vi "DatabaseHand_Element_Get(string).vi"(7 "nd queue":bool, 8 "error in (no error)":errorcluster, 9 "default value":string, 10 "name":string, 11 "Database RefNum in":T1) -> (0 "error out":errorcluster, 1 "type":string, 2 "value":string, 3 "Database RefNum out":T1, 4 "permissions":string="RW", 5 "group":string, 6 "unit":string)   [LabVIEW 2016]
doc: "This VI finds the RefNum of an existing object with the input Name or creates a new object if the Name is not found or Name is unwired or an empty string.\nCopyright 2001 VI Engineering, Inc."
uses:
  DatabaseHand_RefNum.ctl
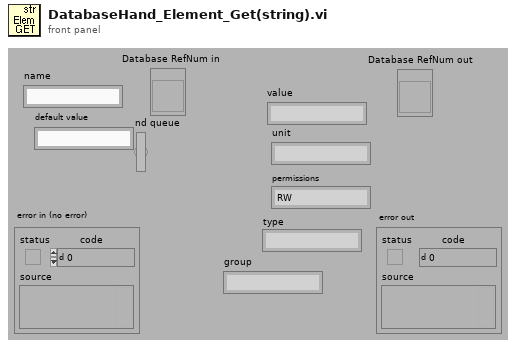
[diagram p1: front panel]
types:
  T1 = typedef "DatabaseHand_RefNum.ctl" = refnum<vi>
  T2 = typedef "DatabaseHand_Element.ctl" = cluster{"name":string, "Database":T3[]}
  T3 = typedef "DatabaseHan_DatabaseElement.ctl" = cluster{"name":string, "value":string, "type":string, "unit":string, "permissions":string, "enqueued":bool, "group":string}
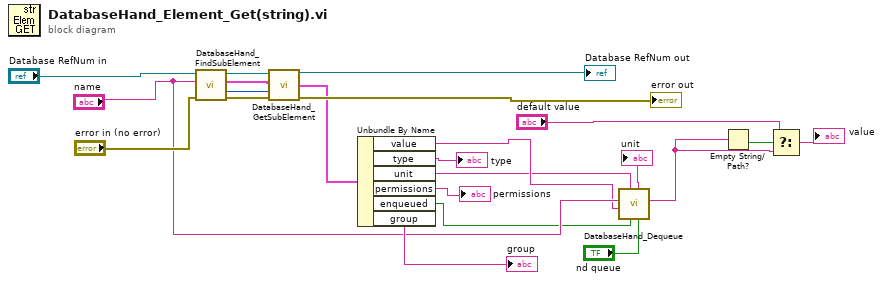
[diagram p0: block diagram]
diagram:
  n1 = call "DatabaseHand_FindSubElement.vi"("error in (no error)"="error in (no error)", "name"="name", "Database RefNum in"="Database RefNum in") -> ("error out"=w18:errorcluster, "index"=w15:i32, "Database"=w19:T2, "Database RefNum out"=w20:T1)  [unwired: 5 out]
  n2 = call "DatabaseHand_GetSubElement.vi"("Database RefNum in"=w20, "Object Data In"=w19, "Index"=w15, "error in (no error)"=w18) -> ("Database RefNum out"=→"Database RefNum out":T1, "Element found"=w14:T3, "error out"=→"error out":errorcluster)  [unwired: 1 in, 8 out]
  n3 = Unbundle By Name(w14) -> ("value"=w5:string, "type"=→"type":string, "unit"=w2:string, "permissions"=→"permissions":string, "enqueued"=w6:bool, "group"=→"group":string)
  n4 = call "DatabaseHand_Dequeue.vi"("non-destructive queue"="nd queue", "queue?"=w6, "unit in"=w2, "value in"=w5, "name"="name") -> ("value out"=w4:string, "unit out"=→"unit":string)  [unwired: 5 out]
  n5 = Empty String/Path?(string/path=w4) -> (empty?=w8:bool)
  n6 = Select(t="default value", s=w8, f=w4) -> (s? t:f=→"value":string)
